vi "ADC SNR_new_param.vi"(8 "error in (no error)":errorcluster, 9 "Sequence parameters":string[][](array[string])=[["Min limit", "Max limit", "Register sheet file", "Register Sheet"], ["", "", "CC2600.xls", "TX_BLE;Trim"], ["Reg write (addr;value)", "Operating frequency [Hz]", "", ""], ["NA", "2.44G", "", ""]], 10 "Run type":i32, 11 "Method parameters":T4={"Dev"={"Do not disturb DUT"=FALSE, "XOSC"=32000000.0, "Board type"="", "EM"="", "Configure tempboard"=TRUE, "Device specific info"=[], "Generic Object"=refnum}, "Method"={"Run type"=1, "Test name"="Current LPM2 4", "Comment"="", "Results folder"="", "AFC"=enum."Off", "Method name"="Current LPM2 4", "Method results"={"Excel brief report"=FALSE, "Spotfire report"=FALSE, "Starfish report"=FALSE}, "Operator"="", "Reference time"=timestamp(0 s since 1904-01-01), "AFC delay"=0.0, "Initialization"=enum."Enabled", "MD5 Sum"="", "HW addon board"=enum."None", "AFC Regsheet"="", "AFC Regfile"=path "", "dummy"=0.0}, "Inst"={"Instr"={"PS1"={"Name"="", "GPIB address"="", "VISA session"=""}, "PS2"={"Name"="", "GPIB address"="", "VISA session"=""}, "TC1"={"Name"="", "GPIB address"="", "VISA session"=""}, "TC2"={"Name"="", "GPIB address"="", "VISA session"=""}, "SA1"={"Name"="", "GPIB address"="", "VISA session"=""}, "SA2"={"Name"="", "GPIB address"="", "VISA session"=""}, "SG1"={"Name"="", "GPIB address"="", "VISA session"=""}, "SG2"={"Name"="", "GPIB address"="", "VISA session"=""}, "SG3"={"Name"="", "GPIB address"="", "VISA session"=""}, "MI1"={"Name"="", "GPIB address"="", "VISA session"=""}, "MI2"={"Name"="", "GPIB address"="", "VISA session"=""}, "SW SA"={"Name"="", "Controller addr"=""}, "SW SG"={"Name"="", "Controller addr"=""}, "MI3"={"Name"="", "GPIB address"="", "VISA session"=""}}, "Switchbox"={"RF Path"=0, "Cal compensation"=enum."TX", "Switchbox gain mode"="", "State"=enum."TX"}, "Instr to control (i.e. SA1)"="Default", "Intrument info string"=""}, "Sequence parameters"=[["Weight", "Min Limit", "Max Limit", "Register Sheet", "", "", "", "", "", "", "", "", ""], ["Vital", "", "1", "LPM2", "", "", "", "", "", "", "", "", ""], ["Resolution", "Reg write (addr;value)", "Chip mode", "Range", "", "", "", "", "", "", "", "", ""], ["u", "NA", "", "auto", "", "", "", "", "", "", "", "", ""]], "Cond"={"Temp logged"=25.0, "VDD1_PS1_6V"=-999.0, "VDD2_PS1_25V"=-999.0, "VDD4_PS2_25V"=-999.0, "VDD3_PS2_6V"=-999.0}, "Meas config"={"X-axis inner loop index"=32000000, "Y-axis outer loop index"=32000000, "X-axis"=[], "Y-axis"=[], "X-axis array req size"=32000000, "Y-axis array req size"=32000000, "Param description"=[], "Use meas clust for reporting"=FALSE, "Parameter index (page)"=0, "X-axis name"="", "Y-axis name"=""}} {"Cond"."VDD3_PS2_6V" format="%.3f"; "Cond"."VDD4_PS2_25V" format="%.3f"; "Cond"."VDD2_PS1_25V" format="%.3f"; "Cond"."VDD1_PS1_6V" format="%.3f"; "Method"."dummy" format="%.1p"; "Method"."AFC delay" format="%.1p"; "Dev"."XOSC" format="%.3p"}) -> (0 "error out":errorcluster, 1 "End method error":T2, 2 "Short Results":string[](array[string])=["0.00", "0.00", "0.00", "0.00"], 3 "Result summary":string[][](array[string])=[["Critical", "Output Power@2405 MHz", "-3", "4", "dBm"], ["Critical", "Output Power@2410 MHz", "-3", "4", "dBm"]])   [LabVIEW 2019]
doc: "[AutoDocStart]Performs crystal accuracy measurements. Measures the offset from ideal frequency. Primarily used for tuning XOSC capacitors and verifying XOSC trims.\n\nSweeping parameters: operating frequency, OSC override value and VDDR level\n\nResults: Offset frequency in ppm[AutoDocEnd]"
uses:
  User Lib/Utilities/Cluster definitions/Method input.ctl
  User Lib/Utilities/Cluster definitions/Device specific info.ctl
  User Lib/Utilities/Controls/Automatic Frequency Compensation types.ctl
  User Lib/Utilities/Controls/Method Reports.ctl
  User Lib/Utilities/Cluster definitions/Method Initialization.ctl
  User Lib/Utilities/Controls/HW addon boards.ctl
  User Lib/Utilities/Cluster definitions/Instr clust.ctl
  User Lib/Utilities/Switchbox control/SwitchBox_State._ENUMctl.ctl
  User Lib/Utilities/Cluster definitions/End method error cluster.ctl
  User Lib/Utilities/Cluster definitions/DUT vdd control.ctl
  User Lib/Utilities/Cluster definitions/DUT VDD4.ctl
  User Lib/Utilities/Cluster definitions/DUT VDD3.ctl
  User Lib/Utilities/Cluster definitions/DUT VDD2.ctl
  User Lib/Utilities/Cluster definitions/DUT VDD1.ctl
  User Lib/Generic chip methods/Classes/Generic_EM/Chameleon/Loki/Loki.lvclass
  <vilib>/Utility/error.llb/Clear Errors.vi
  User Lib/Generic chip methods/Classes/Generic_EM/Chameleon/65nm.lvclass
  C:/Kharon/User Lib/Generic chip methods/Classes/Generic_EM/Generic_EM/Generic_EM.lvclass
  User Lib/Generic chip methods/board_to_chip_type.vi
  User Lib/Generic chip methods/Classes/Get_Class_init.vi
  User Lib/Generic chip methods/Classes/Generic_EM/Generic_EM/Generic_EM.lvclass
panel:
  in  "Tab Control":T1(tab)
  out "Dynamic Parameters":T3={"SNR"=nan, "SNRD"=nan, "THD"=nan, "ENOB (SNRD)"=nan, "SFDR"=nan, "ENOB (SNR)"=nan, "Noise Power"=nan, "Signal power"=nan} {"Signal power" format="%.6f"; "Noise Power" format="%.2f"; "ENOB (SNR)" format="%.2f"; "SFDR" format="%.2f"; "ENOB (SNRD)" format="%.2f"; "THD" format="%.2f"; "SNRD" format="%.2f"; "SNR" format="%.2f"}
  out "ADC samples":u32[](array[numeric])
  out "Output Response [All DUTs]":u32[][](array[numeric])
  out "SNR":dbl
  out "Noise Power":dbl
  out "Signal power":dbl
  out "ENOB (SNR)":dbl
  out "detected Throughput":dbl=200065.4236150998
  # "°C"
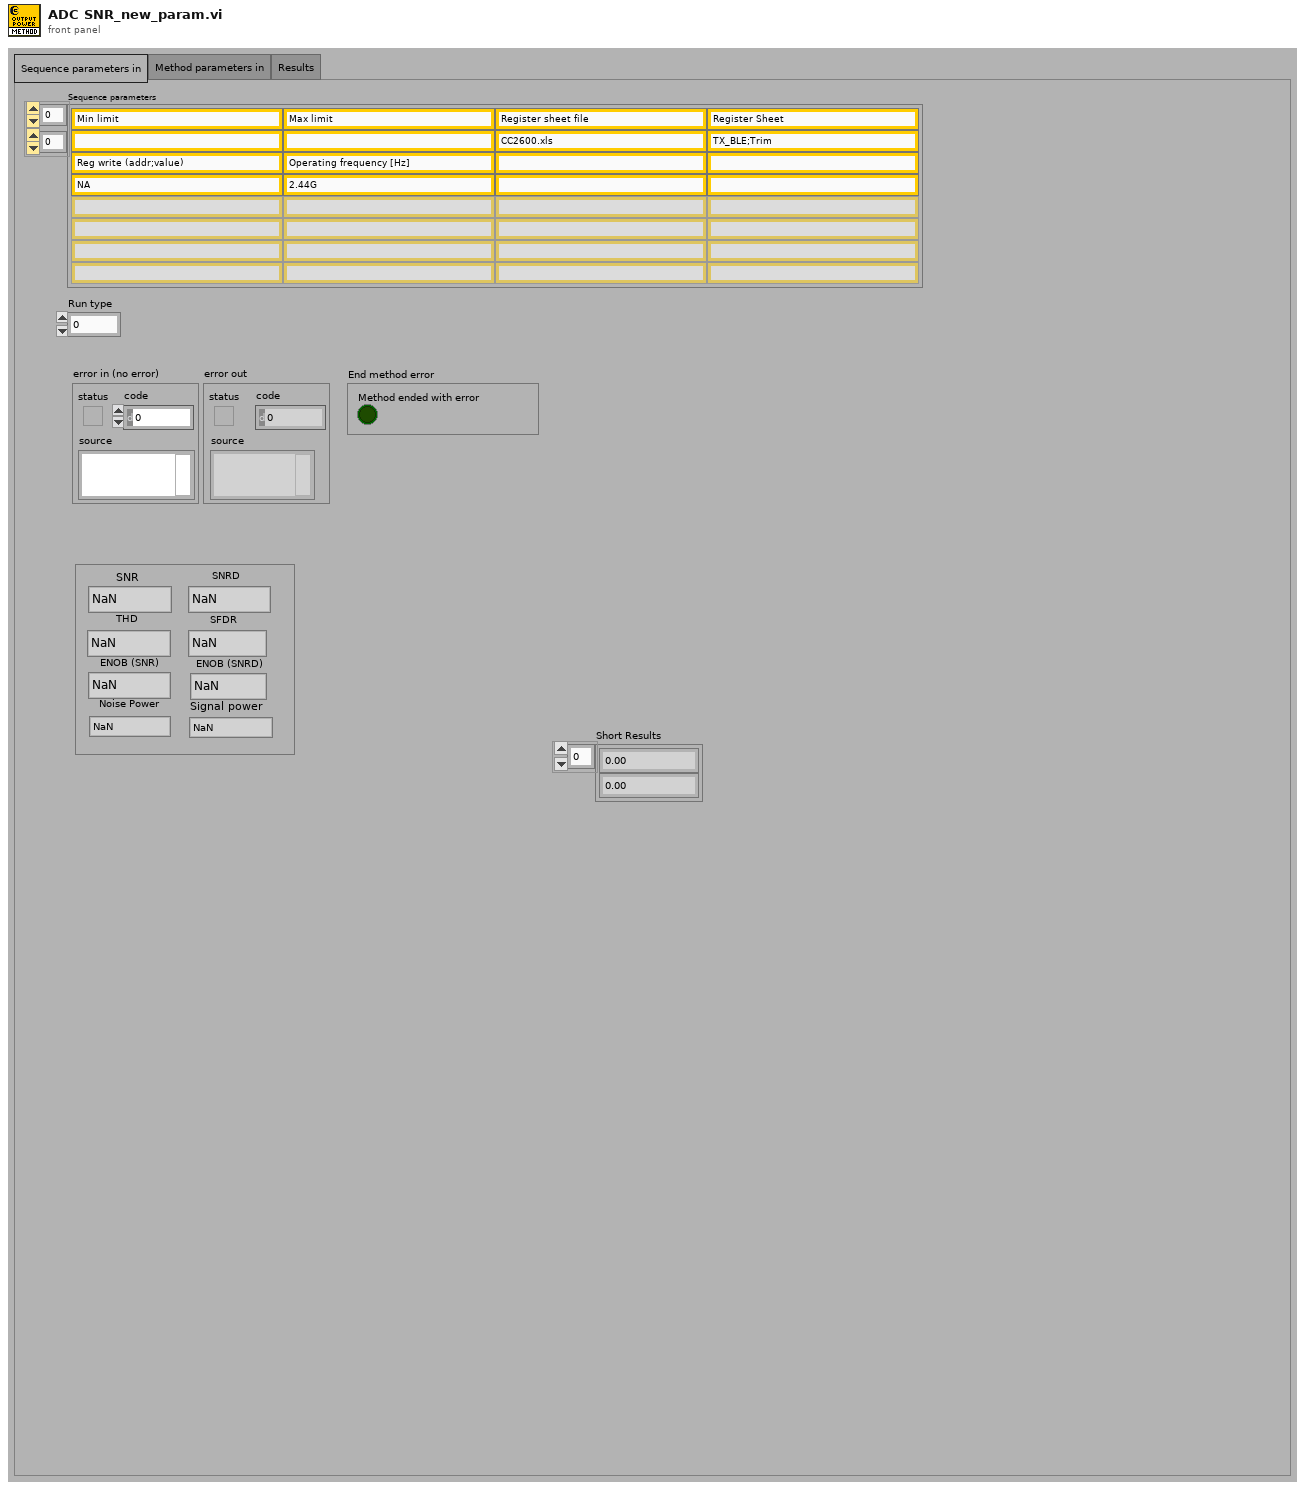
[diagram p1: front panel]
types:
  T1 = enum32{"Sequence parameters in", "Method parameters in", "Results"}
  T2 = typedef "End method error cluster.ctl" = cluster{"Method ended with error":bool}
  T3 = cluster{"SNR":dbl, "SNRD":dbl, "THD":dbl, "ENOB (SNRD)":dbl, "SFDR":dbl, "ENOB (SNR)":dbl, "Noise Power":dbl, "Signal power":dbl}
  T4 = typedef "Method input.ctl" = cluster{"Dev":cluster{"Do not disturb DUT":bool, "XOSC":dbl, "Board type":string, "EM":string, "Configure tempboard":bool, "Device specific info":T5[], "Generic Object":refnum<class>}, "Method":cluster{"Run type":i32, "Test name":string, "Comment":string, "Results folder":string, "AFC":T6, "Method name":string, "Method results":T7, "Operator":string, "Reference time":timestamp, "AFC delay":dbl, "Initialization":T8, "MD5 Sum":string, "HW addon board":T9, "AFC Regsheet":string, "AFC Regfile":path, "dummy":dbl}, "Inst":T10, "Sequence parameters":string[][], "Cond":cluster{"Temp logged":dbl, "VDD1_PS1_6V":dbl, "VDD2_PS1_25V":dbl, "VDD4_PS2_25V":dbl, "VDD3_PS2_6V":dbl}, "Meas config":cluster{"X-axis inner loop index":i32, "Y-axis outer loop index":i32, "X-axis":string[], "Y-axis":string[], "X-axis array req size":i32, "Y-axis array req size":i32, "Param description":string[][], "Use meas clust for reporting":bool, "Parameter index (page)":i32, "X-axis name":string, "Y-axis name":string}}
  T5 = typedef "Device specific info.ctl" = cluster{"EM number":u8, "IP address":string, "Enabled":bool, "Slot no":u8, "RF path":u8, "EM name":string, "Wafer info":string, "AFC frequency ppm":dbl, "Register writes":string[][], "Meas data":string[][][], "Device comment":string}
  T6 = typedef "Automatic Frequency Compensation types.ctl" = enum16{"Off", "Compensate Instrument frequency", "Compensate DUT frequency", "Predictive - Compensate Instrument frequency", "Predictive - Compensate DUT frequency", "Do not skip re-init - Compensate Instrument frequency", "Do not skip re-init - Compensate DUT frequency"}
  T7 = typedef "Method Reports.ctl" = cluster{"Excel brief report":bool, "Spotfire report":bool, "Starfish report":bool}
  T8 = typedef "Method Initialization.ctl" = enum16{"Enabled", "Skip Instr and Device Init", "Enabled with Separate Flash", "Set PS, Device Init and Skip Instr Init", "Skip Device Init"}
  T9 = typedef "HW addon boards.ctl" = enum16{"None", "Current meas 5EM", "Stresstest 10EM"}
  T10 = typedef "Instr clust.ctl" = cluster{"Instr":cluster{"PS1":cluster{"Name":string, "GPIB address":string, "VISA session":refnum<visa-resource-name>}, "PS2":cluster{"Name":string, "GPIB address":string, "VISA session":refnum<visa-resource-name>}, "TC1":cluster{"Name":string, "GPIB address":string, "VISA session":refnum<visa-resource-name>}, "TC2":cluster{"Name":string, "GPIB address":string, "VISA session":refnum<visa-resource-name>}, "SA1":cluster{"Name":string, "GPIB address":string, "VISA session":refnum<visa-resource-name>}, "SA2":cluster{"Name":string, "GPIB address":string, "VISA session":refnum<visa-resource-name>}, "SG1":cluster{"Name":string, "GPIB address":string, "VISA session":refnum<visa-resource-name>}, "SG2":cluster{"Name":string, "GPIB address":string, "VISA session":refnum<visa-resource-name>}, "SG3":cluster{"Name":string, "GPIB address":string, "VISA session":refnum<visa-resource-name>}, "MI1":cluster{"Name":string, "GPIB address":string, "VISA session":refnum<visa-resource-name>}, "MI2":cluster{"Name":string, "GPIB address":string, "VISA session":refnum<visa-resource-name>}, "SW SA":cluster{"Name":string, "Controller addr":string}, "SW SG":cluster{"Name":string, "Controller addr":string}, "MI3":cluster{"Name":string, "GPIB address":string, "VISA session":refnum<visa-resource-name>}}, "Switchbox":cluster{"RF Path":i32, "Cal compensation":enum16{"TX", "RX", "Interferer", "No compensation", "Interferer2"}, "Switchbox gain mode":string, "State":T11}, "Instr to control (i.e. SA1)":string, "Intrument info string":string}
  T11 = typedef "SwitchBox_State._ENUMctl.ctl" = enum16{"TX", "RX", "SP:TX", "SP:RX", "SW:TX", "SW:RX"}
  T12 = cluster{"Fundamental Frequency":dbl, "Sampling Frequncy":dbl, "No of Harmonics":u8, "Window":enum16{"None ", "Hanning", "Hamming", "Blackman-Harris", "Exact Blackman", "Blackman", "Flat Top", "4 Term B-Harris ", "7 Term B-Harris"}, "Blackman (fundamental power) bins)":dbl}
  T13 = typedef "DUT vdd control.ctl" = cluster{"VDD4 config":T14, "VDD3 config":T15, "VDD2 config":T16, "VDD1 config":T17}
  T14 = typedef "DUT VDD4.ctl" = u16
  T15 = typedef "DUT VDD3.ctl" = u16
  T16 = typedef "DUT VDD2.ctl" = u16
  T17 = typedef "DUT VDD1.ctl" = u16
  T18 = enum32{"NI Card Settings", "Memory Read Setting", "DC Capture", "ADC Ramp", "ADC Sine", "SNR", "Cap Calibration"}
  T19 = enum32{"Read from Memory", "Read .dat file", "NI Card Capture", "None"}
  T20 = typedef "TFW ResponseData.ctl" = cluster{"errorCode":u32, "executionTime":u32, "processedCmdWord":u32, "responsePar":u32[], "actionCode":u32, "cmdStatus":u16}
  T21 = cluster{"Path to Save plot":path, "Path to Raw Data plot":path}
  T22 = cluster{"Save INL/DNL Plot(Ramp)":bool, "Save SNR Plot":bool, "Save INL/DNL Plot(Sine)":bool, "Save INL/DNL Raw Data(Ramp)":bool, "Save SNR Raw Data":bool, "Save INL/DNL Raw Data(Sine)":bool, "Save DC Raw data":bool, "Save  Raw Data(Sine)":bool}
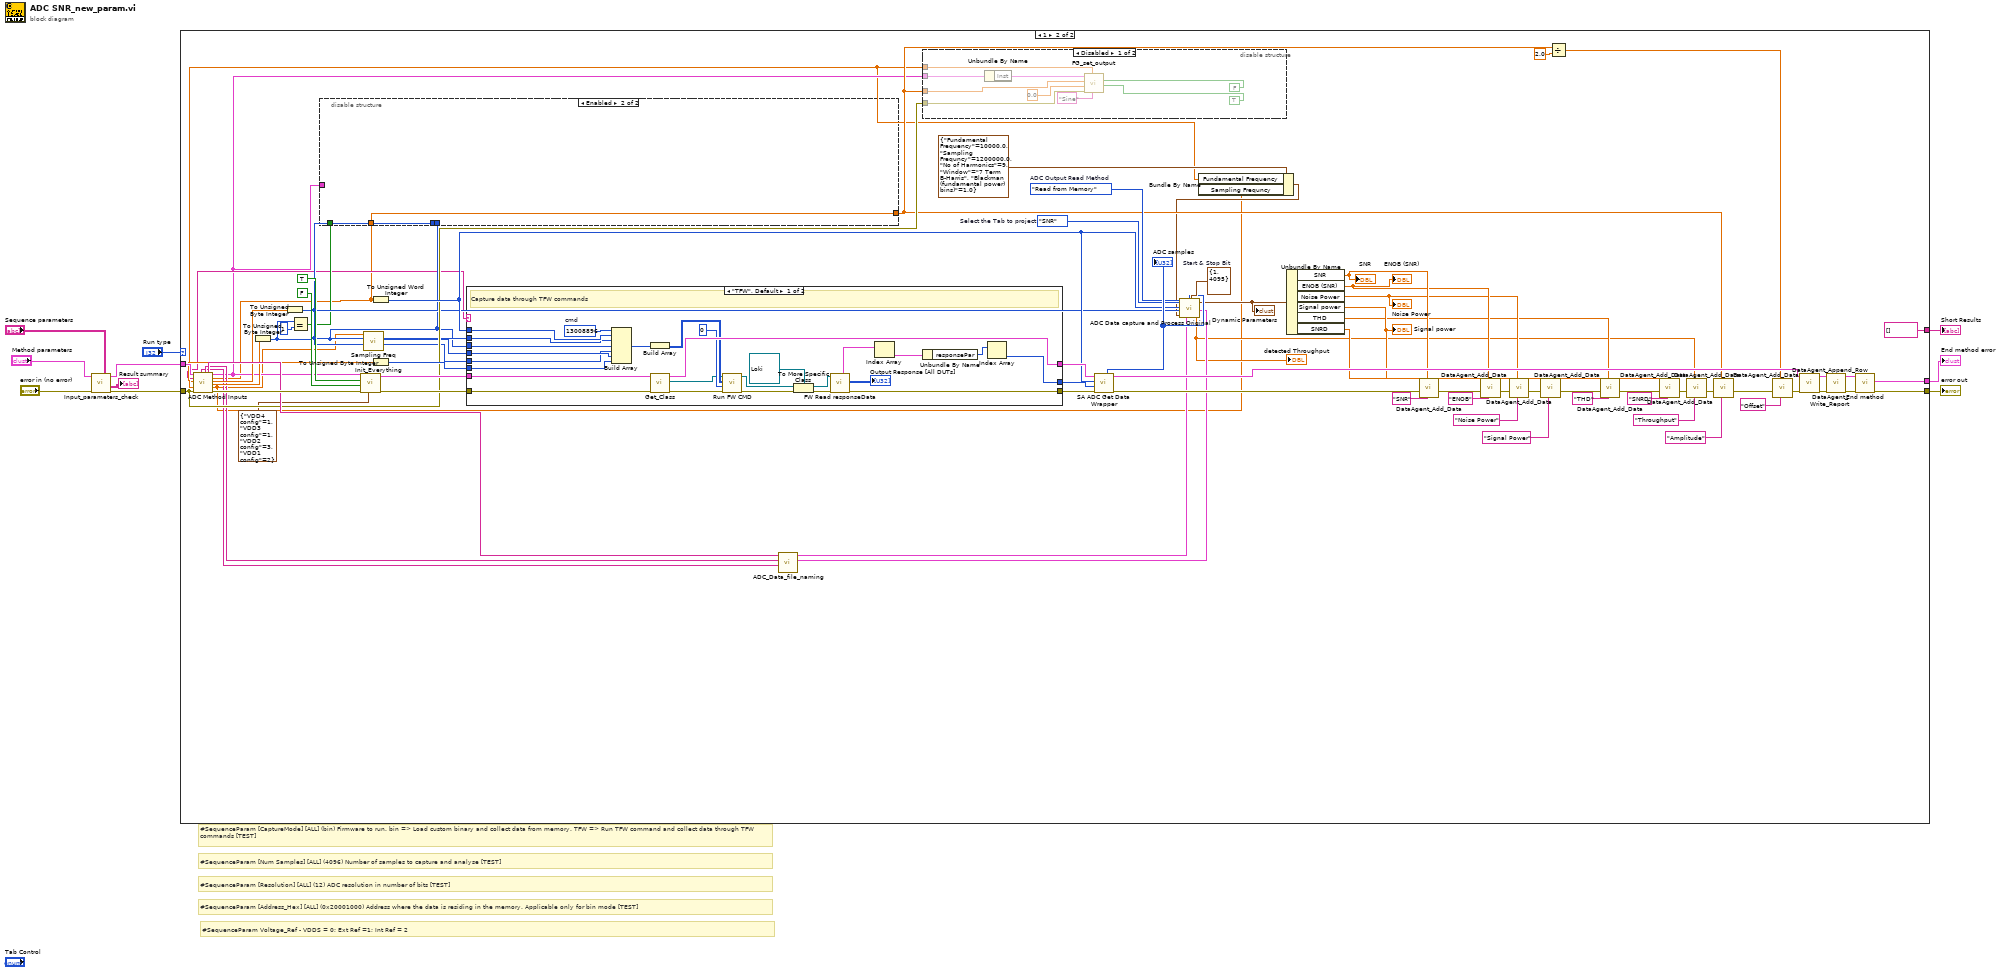
[diagram p0: block diagram]
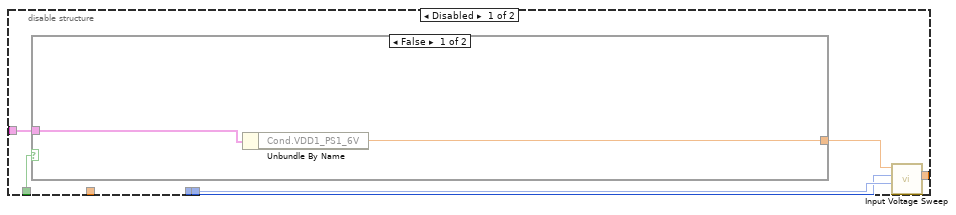
[diagram p3: hidden frame]
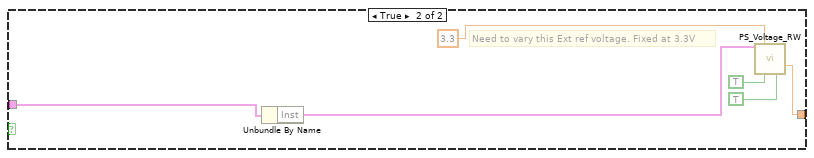
[diagram p4: hidden frame]
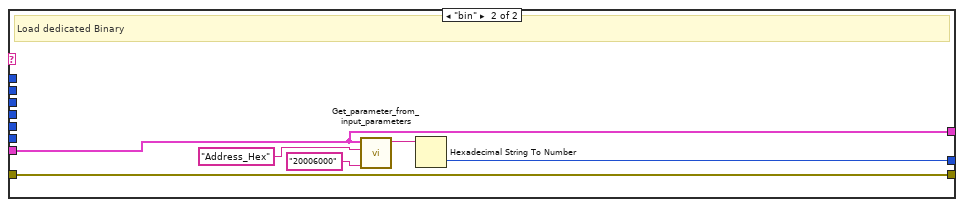
[diagram p6: hidden frame]
diagram:
  # "#SequenceParam Voltage_Ref - VDDS = 0; Ext Ref =1; Int Ref = 2"
  # "#SequenceParam [Num Samples] [ALL] (4096) Number of samples to capture and analyse [TEST]"
  # "#SequenceParam [CaptureMode] [ALL] (bin) Firmware to run. bin => Load custom binary and collect data from memory. TFW => Run TFW command and collect data through TFW commands [TEST]"
  # "#SequenceParam [Address_Hex] [ALL] (0x20001000) Address where the data is residing in the memory. Applicable only for bin mode [TEST]"
  # "#SequenceParam [Resolution] [ALL] (12) ADC resolution in number of bits [TEST]"
  n1 = call "Input_parameters_check.vi"("Sequence parameters"="Sequence parameters", "error in"="error in (no error)", "Method cluster in"="Method parameters") -> ("error out"=w9:errorcluster, "Result summary"=→"Result summary":string[][], "Method cluster out"=w5:T4)  [unwired: 6 in]
  n2 = case shown="1" "Run type" {
    tunnel: w9 -> [w11 w40]
    tunnel: [w11 w87] -> w10
    tunnel: w5 -> [_ w25]
    tunnel: [_ w86] -> w4
    tunnel: [_ string[] []] -> w1
    frame 0, Default {
      # "Run type 0 is only for formatting the result summary"
    }
    frame 1 {
      w49 = cluster{"Start":i32, "Stop":i32} {"Start"=1, "Stop"=4095}  # Start & Stop Bit
      w42 = T18."SNR"  # Select the Tab to project
      w43 = T19."Read from Memory"  # ADC Output Read Method
      n3 = call "ADC Method Inputs.vi"("Method cluster in"=w25, "error in (no error)"=w40) -> ("Capture Mode"=w20:string, "Signal Freq"=w14:dbl, "ADC Chnl No."=w21:dbl, "Sampling Freq String"=w18:string, "Resolution String"=w19:string, "Voltage Ref String"=w50:string, "Method cluster out"=w17:T4, "Num Samples"=w12:dbl, "Resolution"=w24:dbl, "Voltage Ref"=w23:dbl, "Sampling Freq"=w13:dbl, "error out"=w85:errorcluster)  [unwired: 5 in, 1 out]
      n4 = To Unsigned Byte Integer(number=w23) -> (unsigned 8bit integer=w27:u8)
      n5 = To Unsigned Byte Integer(number=w24) -> (unsigned 8bit integer=w30:u8)
      n6 = Equal?(x=w27, y=u8 1) -> (x = y?=w29:bool)
      n7 = disable-structure shown="Enabled" {
        disable-tunnel: [w93 w102] -> w31
        disable-tunnel: w30 -> [w92 _]
        disable-tunnel: w29 -> [w91 _]
        disable-tunnel: w27 -> [w90 _]
        disable-tunnel: w17 -> [w88 _]
        disable-tunnel: w12 -> [_ w102]
        frame Disabled {
          n8 = case shown="False" w91 {
            tunnel: [w94 w98] -> w89
            tunnel: w88 -> [w95 w97]
            frame False {
              n9 = Unbundle By Name(w95) -> ("Cond.VDD1_PS1_6V"=w94:dbl)
            }
            frame True {
              # "Need to vary this Ext ref voltage. Fixed at 3.3V"
              n10 = Unbundle By Name(w97) -> ("Inst"=w96:T10)
              n11 = call "PS_Voltage_RW.vi"("InstrCluster in"=w96, "Set Voltage"=3.3, "Off (F)                         On (T)"=TRUE, "Read (F)                      Write (T)"=TRUE) -> ("Output Voltage"=w98:dbl)  [unwired: 9 in, 2 out]
            }
          }
          n12 = call "Input Voltage Sweep.vi"("Resolution"=w92, "Voltage Ref"=w90, "VDDS"=w89) -> ("High Voltage"=w93:dbl)  [unwired: 8 in]
        }
        frame Enabled {
        }
      }
      n13 = call "Init_Everything.vi"("VDD config"=T13 {"VDD4 config"=1, "VDD3 config"=1, "VDD2 config"=3, "VDD1 config"=2}, "error in"=w85, "Support current measurement?"=FALSE, "Override VDD Config"=TRUE, "Method cluster In"=w17) -> ("error out"=w82:errorcluster, "Method cluster out"=w81:T4)  [unwired: 3 in, 2 out]
      n14 = call "Sampling Freq.vi"("Resolution"=w30, "Voltage Ref"=w27, "Sampling Freq"=w13) -> ("LGPT Count"=w22:u16, "SCOMP"=w39:u16)  [unwired: 7 in]
      n15 = To Unsigned Word Integer(number=w12) -> (unsigned 16bit integer=w41:u16)
      n16 = To Unsigned Byte Integer(number=w21) -> (unsigned 8bit integer=w51:u8)
      n17 = case shown="\"TFW\", Default" w20 {
        tunnel: [w137 w138] -> w77
        tunnel: [w130 w143] -> w76
        tunnel: w82 -> [w129 w143]
        tunnel: w81 -> [w136 w138]
        tunnel: [w117 w139] -> w75
        tunnel: w41 -> [w133 _]
        tunnel: w30 -> [w116 _]
        tunnel: w39 -> [w115 _]
        tunnel: w51 -> [w114 _]
        tunnel: w27 -> [w113 _]
        tunnel: w22 -> [w112 _]
        frame "TFW", Default {
          w134 = u32 13008896  # cmd
          # "Capture data through TFW commands"
          n18 = Build Array(w134, w133, w116, w113, w112, w115, w114) -> (w132:u32[])
          n19 = Build Array(w132) -> (w131:u32[][])
          n20 = call "Get_Class.vi"("error in (no error)"=w129, "Method cluster in"=w136) -> ("error out"=w127:errorcluster, "Class Out"=w126:refnum<class "Generic_EM.lvclass">, "Method cluster out"=w137:T4)  [unwired: 6 in, 1 out]
          n21 = call-dynamic "Run FW CMD.vi"("error in (no error)"=w127, "Handler"=u8 0, "cmdBuf"=w131, "Generic_EM in"=w126) -> ("error out"=w122:errorcluster, "Generic_EM out"=w125:refnum<class "Generic_EM.lvclass">)  [unwired: 6 in]
          n22 = To More Specific Class(target class=refnum<class "Loki.lvclass"> refnum ("Loki in"), reference=w125, error in=w122) -> (specific class reference=w123:refnum<class "Loki.lvclass">, error out=w121:errorcluster)
          n23 = call "FW Read responseData.vi"("error in (no error)"=w121, "Loki in"=w123) -> ("error out"=w130:errorcluster, "Output Response [All DUTs]"=→"Output Response [All DUTs]":u32[][], "Response"=w119:T20[])  [unwired: 6 in, 1 out]
          n24 = Index Array(array=w119) -> (element=w120:T20)  [unwired: 1 in]
          n25 = Unbundle By Name(w120) -> ("responsePar"=w118:u32[])
          n26 = Index Array(array=w118) -> (element=w117:u32)  [unwired: 1 in]
        }
        frame "bin" {
          # "Load dedicated Binary"
          n27 = call "Get_parameter_from_input_parameters.vi"("Default value (used if not specified on Front Panel)"="20006000", "Parameter name"="Address_Hex" ("SA_ param name"), "Method cluster (if input param empty)"=w138) -> ("value as String"=w142:string)  [unwired: 2 in, 6 out]
          n28 = Hexadecimal String To Number(string=w142) -> (number=w139:u32)  [unwired: 2 in, 1 out]
        }
      }
      n29 = call "ADC_Data_file_naming.vi"("Sampling Freq String"=w18, "Resolution String"=w19, "Voltage Ref String"=w50) -> ("path to save"=w45:T21, "Save data"=w47:T22)  [unwired: 7 in]
      n30 = disable-structure shown="Disabled" {
        disable-tunnel: w40 -> [w106 _]
        disable-tunnel: w31 -> [w105 _]
        disable-tunnel: w17 -> [w104 _]
        disable-tunnel: w14 -> [w103 _]
        frame Disabled {
          n31 = Unbundle By Name(w104) -> ("Inst"=w111:T10)
          n32 = call "FG_set_output.vi"("High impedance (T)"=TRUE, "Invert output"=FALSE, "Function (DC, Sine, Square, Triangle, Ramp up, Ramp down, Pulse)"="Sine", "Frequency [Hz]"=w103, "error in"=w106, "Low voltage"=0.0, "High voltage (or DC)"=w105, "InstrCluster in"=w111) -> ()  [unwired: 2 in, 2 out]
        }
        frame Enabled {
        }
      }
      n33 = call "SA ADC Get Data Wrapper.vi"("error in"=w76, "Data Address"=w75, "Num Samples"=w41, "Method cluster in"=w77) -> ("error out"=w79:errorcluster, "output cluster"=w78:T4, "ADC samples"=w48:u32[])  [unwired: 2 in, 3 out]
      "ADC samples" <- w48
      n34 = Bundle By Name(cluster=T12 {"Fundamental Frequency"=10000.0, "Sampling Frequncy"=1200000.0, "No of Harmonics"=9, "Window"=enum."7 Term B-Harris", "Blackman (fundamental power) bins)"=1.0} ("Inputs for Dyanmic para"), "Fundamental Frequency"=w14, "Sampling Frequncy"=w13) -> (w15:T12)
      n35 = call "ADC Data capture and Process Original.vi"("ADC Output Read Method"=w43, "Select the Tab to project"=w42, "No.of samples(SNR)"=w41, "Resolution"=w30, "Inputs for Dyanmic para"=w15, "Save data"=w47, "Waveform"=w48, "Start & Stop Bit"=w49, "path to save"=w45) -> ("detected Throughput"=w44:dbl, "Dynamic Parameters"=w46:T3)  [unwired: 12 in, 5 out]
      "Dynamic Parameters" <- w46
      "detected Throughput" <- w44
      n36 = Unbundle By Name(w46) -> ("SNR"=w67:dbl, "ENOB (SNR)"=w66:dbl, "Noise Power"=w57:dbl, "Signal power"=w56:dbl, "THD"=w55:dbl, "SNRD"=w54:dbl)
      "SNR" <- w67
      "Noise Power" <- w57
      "Signal power" <- w56
      "ENOB (SNR)" <- w66
      n37 = call "DataAgent_Add_Data.vi"("ColumnName"="SNR" ("Default Value"), "Data"=w67, "error in (no error)"=w79) -> ("error out"=w71:errorcluster)  [unwired: 8 in]
      n38 = call "DataAgent_Add_Data.vi"("ColumnName"="ENOB" ("Default Value"), "Data"=w66, "error in (no error)"=w71) -> ("error out"=w65:errorcluster)  [unwired: 8 in]
      n39 = call "DataAgent_Add_Data.vi"("ColumnName"="Noise Power", "Data"=w57, "error in (no error)"=w65) -> ("error out"=w64:errorcluster)  [unwired: 8 in]
      n40 = call "DataAgent_Add_Data.vi"("ColumnName"="Signal Power", "Data"=w56, "error in (no error)"=w64) -> ("error out"=w59:errorcluster)  [unwired: 8 in]
      n41 = Divide(x=w31, y=2.0) -> (x/y=w34:dbl)
      n42 = call "DataAgent_Add_Data.vi"("ColumnName"="THD", "Data"=w55, "error in (no error)"=w59) -> ("error out"=w58:errorcluster)  [unwired: 8 in]
      n43 = call "DataAgent_Add_Data.vi"("ColumnName"="SNRD", "Data"=w54, "error in (no error)"=w58) -> ("error out"=w53:errorcluster)  [unwired: 8 in]
      n44 = call "DataAgent_Add_Data.vi"("ColumnName"="Throughput", "Data"=w44, "error in (no error)"=w53) -> ("error out"=w32:errorcluster)  [unwired: 8 in]
      n45 = call "DataAgent_Add_Data.vi"("ColumnName"="Amplitude", "Data"=w31, "error in (no error)"=w32) -> ("error out"=w35:errorcluster)  [unwired: 8 in]
      n46 = call "DataAgent_Add_Data.vi"("ColumnName"="Offset", "Data"=w34, "error in (no error)"=w35) -> ("error out"=w36:errorcluster)  [unwired: 8 in]
      n47 = call "DataAgent_Append_Row.vi"("error in (no error)"=w36, "Method cluster in"=w78) -> ("error out"=w73:errorcluster, "Method cluster out"=w74:T4)  [unwired: 8 in]
      n48 = call "DataAgent_Write_Report.vi"("error in (no error)"=w73, "Method cluster in"=w74) -> ("error out"=w84:errorcluster, "Method cluster out"=w83:T4)  [unwired: 8 in]
      n49 = call "End method.vi"("error in"=w84, "Method cluster in"=w83) -> ("error out"=w87:errorcluster, "End method error"=w86:T2)  [unwired: 7 in, 1 out]
    }
  }
  "error out" <- w10
  "End method error" <- w4
  "Short Results" <- w1
